vi "integrate_data view.vi"(8 "Y-column names":string[](array[string])=["col0"], 10 "column extension":string[](array[string])=["SCM1_2020Aug_AC.008.txt"], 11 "Graph array":cluster{"output":dbl[], "output":dbl[]}[](array[cluster])=[{"output"=array[591 elements], "output"=array[591 elements]}]) -> ()   [LabVIEW 2024]
uses:
  <vilib>/Analysis/2dsp.llb/Integral Method.ctl
  <vilib>/Analysis/1siggen.llb/Ramp Pattern by Samples.vi
  <vilib>/Analysis/NI_AALBase.lvlib
  <vilib>/gmath/NI_Gmath.lvlib
  <vilib>/Analysis/NI_AALPro.lvlib
panel:
  out "error code":i32
  out "bkg and subtracted data":cluster{"xi used":dbl[], "Integral X":dbl[]}[](graph)
  in  "remove bkg":bool=TRUE
  in  "Bbkg final":dbl=5.0 format="%.2f"
  in  "Bbkg initial":dbl=4.0 format="%.2f"
  in  "poly. order":i32=2
  in  "bkg removal method":enum16{"polynomial", "Cheby poly"}(ring)
  in  "integration method":T1=1 items=["Trapezoidal Rule", "Simpson's Rule", "Simpson's 3/8 Rule", "Bode Rule"]
  in  "export":T2(ring)=enum."write to clipboard"
  out "raw data/bkg":T3(graph)
  in  "interpol. method":i32(ring)=2 items=["nearest", "linear", "spline", "cubic Hermite", "Lagrange"]
  in  "stop":bool
  in  "use variables":bool
  in  "Interpolation #":i32=5000
  in  "export data":bool
  in  "smoothing factor":i32=1
  in  "final":dbl=5.0 format="%.2f"
  in  "init":dbl format="%.2f"
  out "integrated":cluster{"xi used":dbl[], "Integral X":dbl[]}[](graph)
  in  "variable":string="4.2\n3.5\n3"
  # "(0) Data are clipped defined by the 'init' and 'final'.\n(1) Boxcar averaging (use 'smoothing factor' for adjustment)\n(3) Background removal if necessary. Background removal is done by polynomial (normal or Chebychev).\n            i) fitting is done for the range given by 'Bbkg init' and 'Bbkg final'.\n            ii) the background curve is extended to the whole data range."
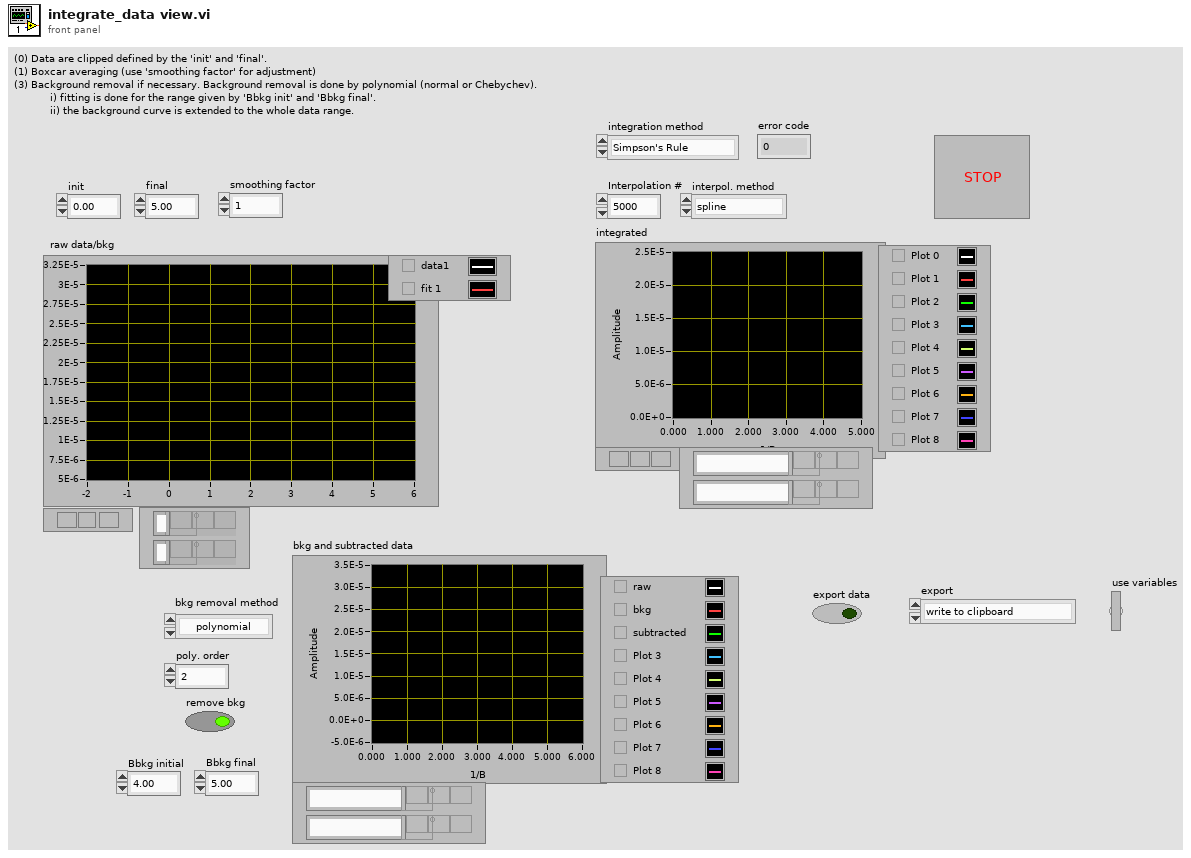
[diagram p1: front panel]
types:
  T1 = typedef "NI_AALPro.lvlib/Integral Method.ctl" = i32
  T2 = enum16{"Save as Ascill file", "write to clipboard", "write to Igor ITX file"}
  T3 = cluster{"Ramp Pattern":dbl[], "Power Spectrum":dbl[]}[]
  T4 = enum16{"Save as Ascill file", "write to clipboard", "do not export"}
  T5 = cluster{"all rows":dbl[], "extended data":dbl[]}[]
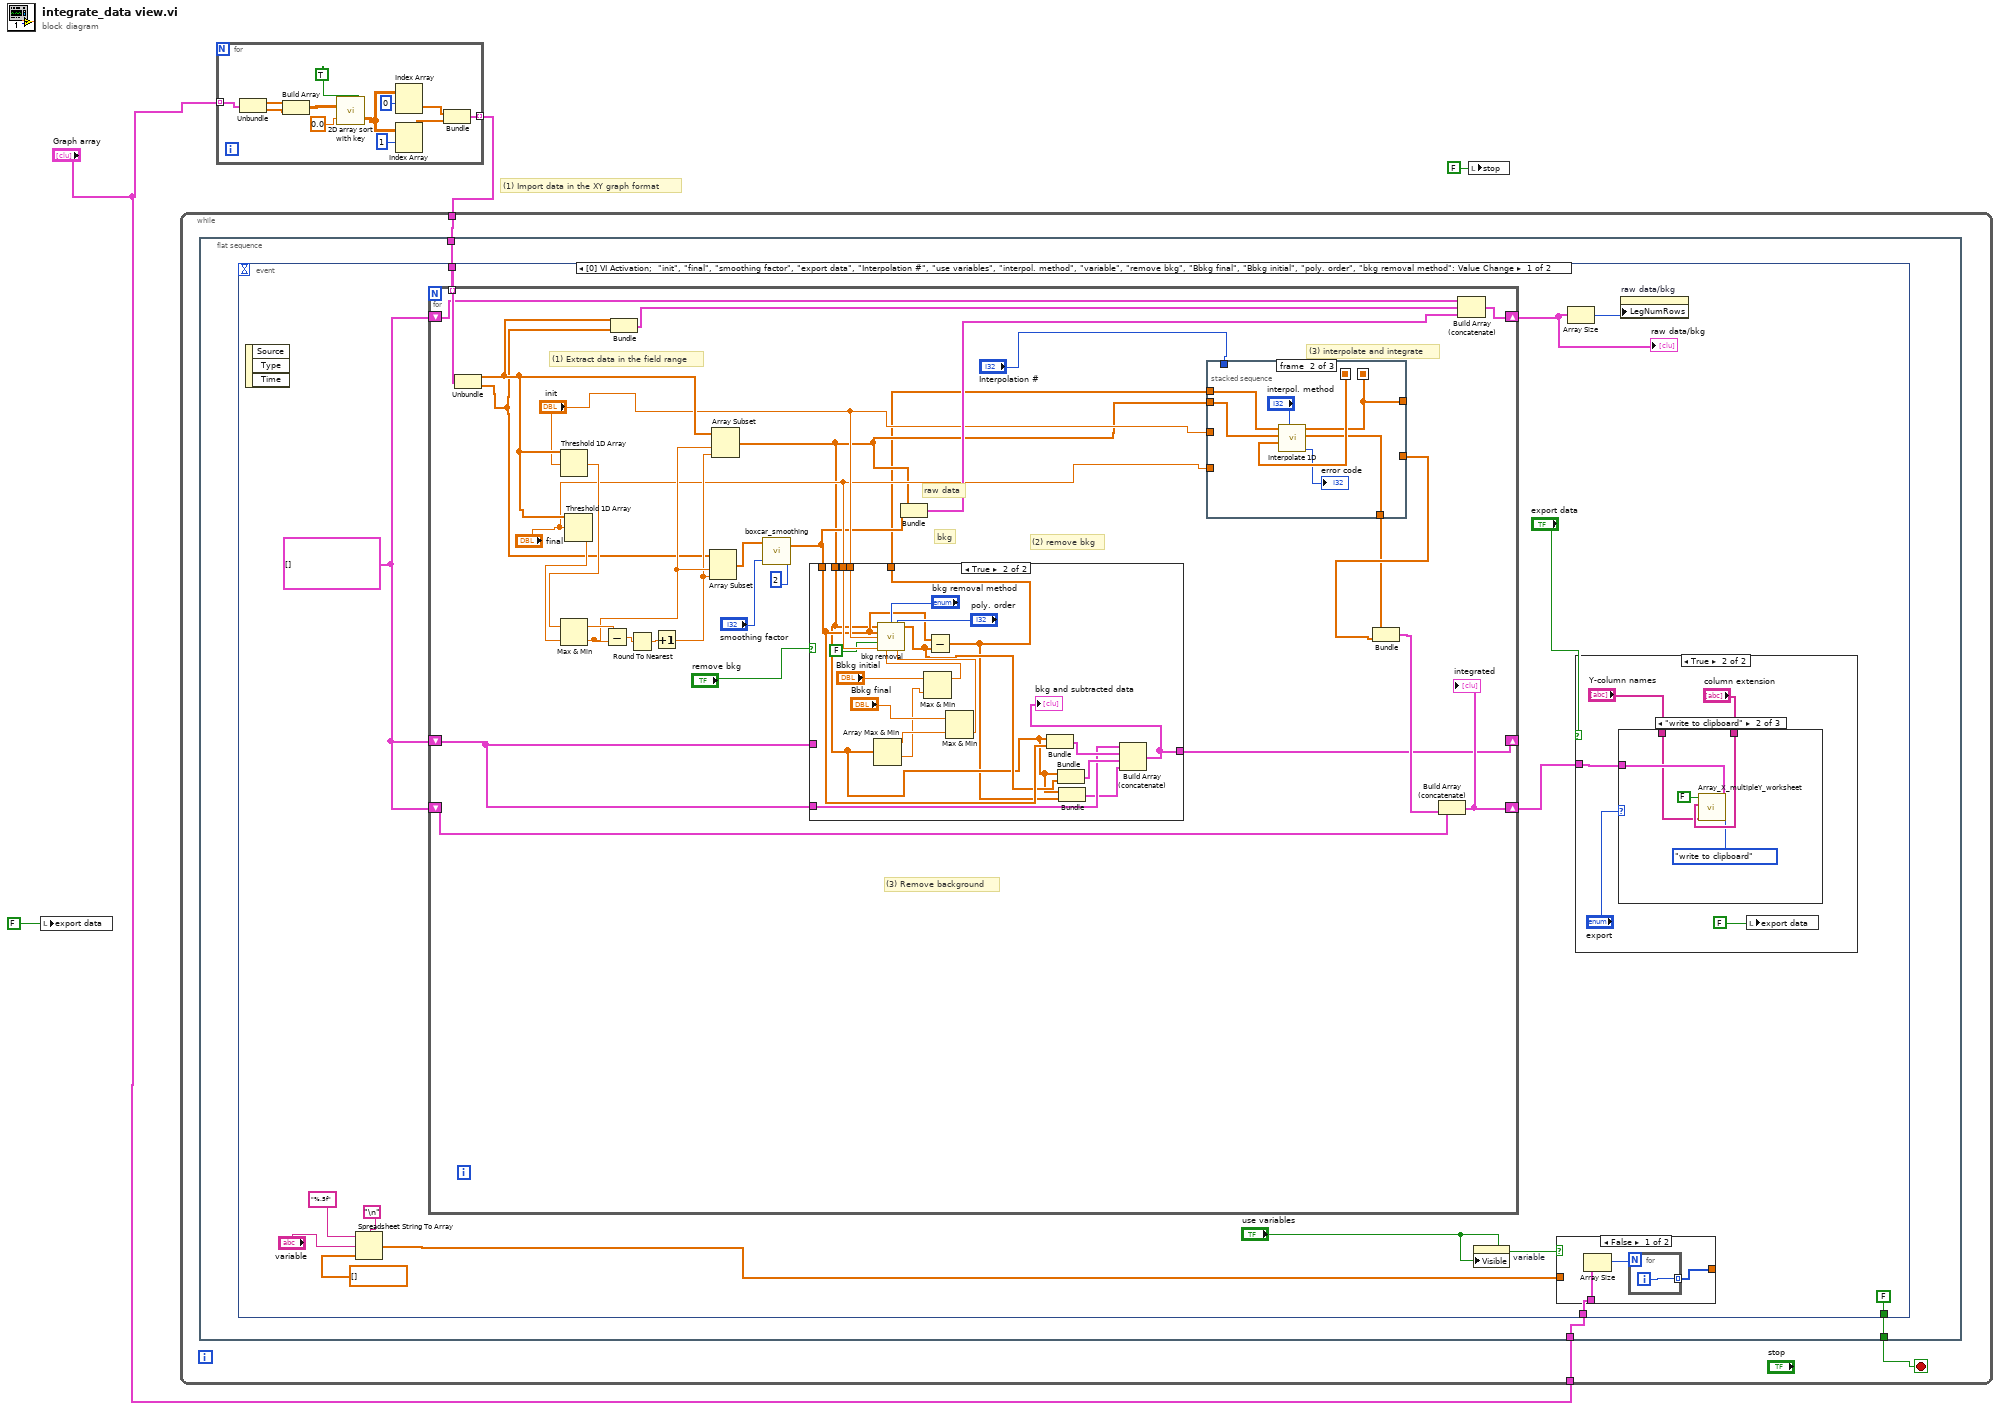
[diagram p0: block diagram]
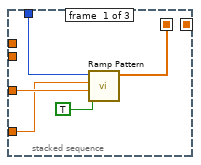
[diagram p4: hidden frame]
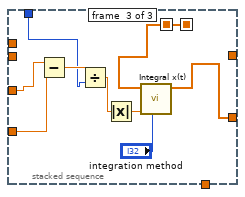
[diagram p5: hidden frame]
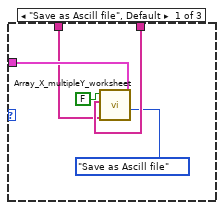
[diagram p7: hidden frame]
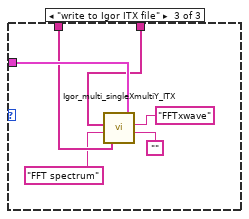
[diagram p8: hidden frame]
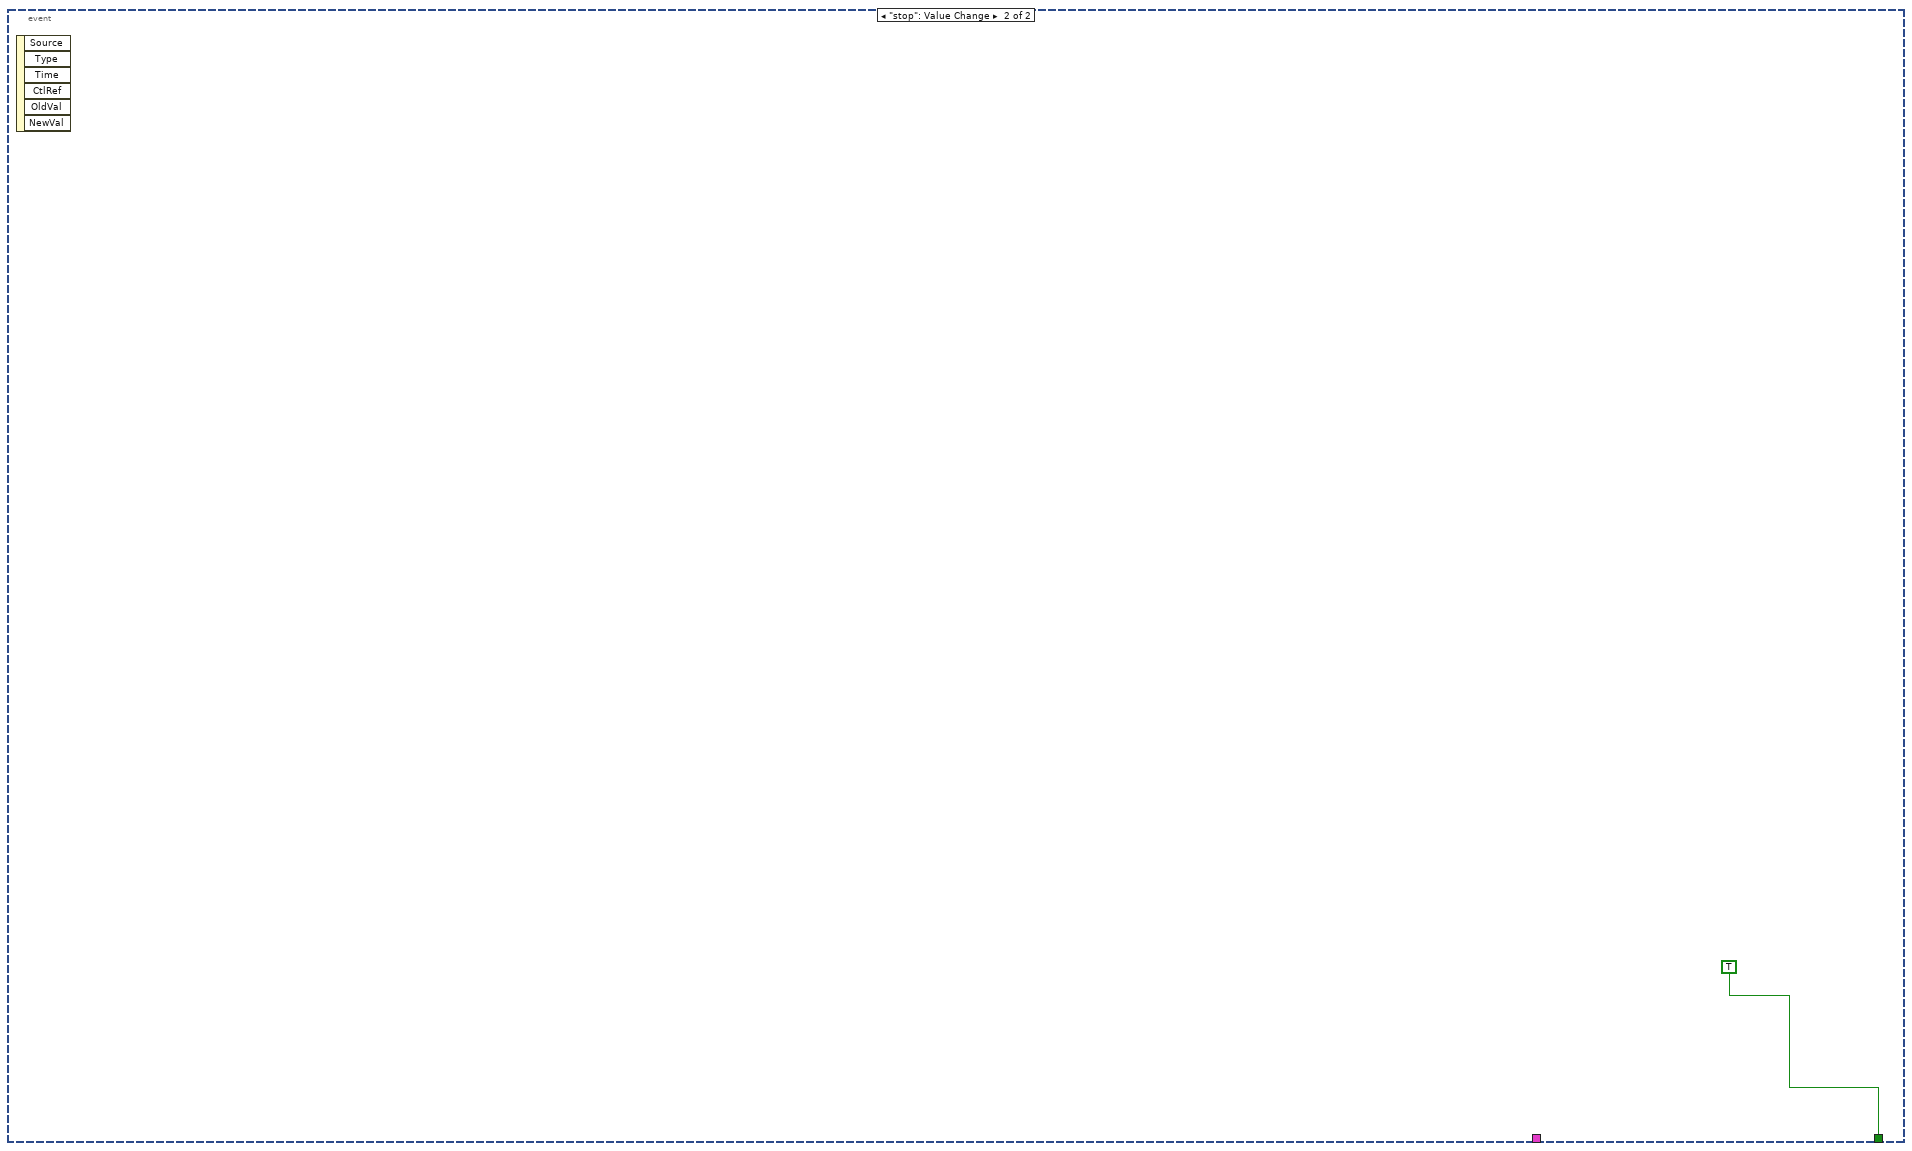
[diagram p9: hidden frame]
diagram:
  # "(1) Import data in the XY graph format"
  n1 = local write "export data"(FALSE ("export spectrum")) -> ()
  n2 = for {
    tunnel: "Graph array" -> [w16] mode=indexing
    tunnel: [w5] -> w3 mode=indexing
    n3 = Unbundle(w16) -> ("output"=w14:dbl[], "output"=w13:dbl[])
    n4 = Build Array(w14, w13) -> (w12:dbl[][])
    n5 = call "2D array sort with key.vi"("ascending"=TRUE, "key row"=0.0, "input"=w12) -> ("output"=w10:dbl[][])
    n6 = Index Array(array=w10, index (row)=0) -> (element=w7:dbl[])  [unwired: 1 in]
    n7 = Index Array(array=w10, index (row)=1) -> (element=w6:dbl[])  [unwired: 1 in]
    n8 = Bundle("output"=w7, "output"=w6) -> (w5:cluster{"output":dbl[], "output":dbl[]})  [unwired: 1 in]
  }
  n9 = while {
    tunnel: w3 -> [w19]
    tunnel: "Graph array" -> [w18]
    stop <- w17 stop-if-true
    n10 = flat-sequence {
      tunnel: w19 -> [w22]
      tunnel: w18 -> [w21]
      tunnel: [w20] -> w17
      frame #0 {
        n11 = event shown="[0] VI Activation;  \"init\", \"final\", \"smoothing factor\", \"export data\", \"Interpolation #\", \"use variables\", \"interpol. method\", \"variable\", \"remove bkg\", \"Bbkg final\", \"Bbkg initial\", \"poly. order\", \"bkg removal method\": Value Change" {
          selector: _ -> [_ _]
          dyn-events: _ -> [_ _]
          timeout: _ -> [_ _]
          tunnel: w22 -> [w31 _]
          tunnel: w21 -> [w29 _]
          tunnel: [FALSE ("stop (press twice)") TRUE ("stop (press twice)")] -> w20
          event VI Activation; "init", "final", "smoothing factor", "export data", "Interpolation #", "use variables", "interpol. method", "variable", "remove bkg", "Bbkg final", "Bbkg initial", "poly. order", "bkg removal method": Value Change {
            w23 = cluster{"all rows":sgl[], "all rows":sgl[]}[] []
            n12 = event-data() -> ()  [unwired: 1 in, 3 out]
            n13 = Spreadsheet String To Array(delimiter (Tab)="\n", format string="%.5f", spreadsheet string="variable", array type (2D Dbl)=dbl[] []) -> (array=w30:dbl[])
            n14 = for {
              shift-right: [w64] -> w24
              shift-left: w23 -> [w71]
              tunnel: w31 -> [w63] mode=indexing
              shift-right: [w61] -> w28
              shift-left: w23 -> [w60]
              shift-right: [w45] -> _
              shift-left: w23 -> [w44]
              # "(2) remove bkg"
              # "(3) interpolate and integrate"
              # "(3) Remove background"
              # "(1) Extract data in the field range"
              # "bkg"
              # "raw data"
              n15 = Unbundle(w63) -> ("output"=w59:dbl[], "output"=w56:dbl[])
              n16 = Threshold 1D Array(2:"init", 3:w59) -> (0:w70:dbl)  [unwired: 1 in]
              n17 = Threshold 1D Array(2:"final", 3:w59) -> (0:w69:dbl)  [unwired: 1 in]
              n18 = Max & Min(x=w70, y=w69) -> (max(x,y)=w68:dbl, min(x,y)=w66:dbl)
              n19 = Subtract(x=w68, y=w66) -> (x-y=w67:dbl)
              n20 = Bundle("output"=w59, "output"=w56) -> (w58:cluster{"output":dbl[], "output":dbl[]})  [unwired: 1 in]
              n21 = Round To Nearest(number=w67) -> (nearest integer value=w72:dbl)
              n22 = Increment(x=w72) -> (x+1=w65:dbl)
              n23 = Array Subset(array=w56, index=w66, length=w65) -> (w55:dbl[])
              n24 = Array Subset(array=w59, index=w66, length=w65) -> (w43:dbl[])
              n25 = call "boxcar_smoothing.vi"("iteration Number"=2, "smooth factor"="smoothing factor", "raw data"=w55) -> ("smoothed"=w46:dbl[])  [unwired: 1 in]
              n26 = case shown="True" "remove bkg" {
                tunnel: w43 -> [_ w77]
                tunnel: w46 -> [w74 w83]
                tunnel: "init" -> [_ w94]
                tunnel: "final" -> [_ w93]
                tunnel: [w74 w76] -> w42
                tunnel: [w73 w78] -> w45
                tunnel: w44 -> [_ w79]
                tunnel: w44 -> [w73 _]
                frame False {
                }
                frame True {
                  n27 = Array Max & Min(array=w77) -> (max value=w88:dbl, min value=w87:dbl)  [unwired: 2 out]
                  n28 = Max & Min(x="Bbkg initial", y=w87) -> (max(x,y)=w84:dbl)  [unwired: 1 out]
                  n29 = Max & Min(x="Bbkg final", y=w88) -> (min(x,y)=w85:dbl)  [unwired: 1 out]
                  n30 = call "bkg removal.vi"("Bfield"=w77, "bkg removal method"="bkg removal method", "poly. order"="poly. order", "Data"=w83, "B initial"=w94, "inverse"=FALSE, "B final"=w93, "Bbkg initial"=w84, "Bbkg final"=w85) -> ("extended data"=w82:dbl[])  [unwired: 4 in, 2 out]
                  n31 = Subtract(x=w83, y=w82) -> (x-y=w76:dbl[])
                  n32 = Bundle(w77, "smoothed"=w83) -> (w81:cluster{dbl[], "smoothed":dbl[]})  [unwired: 1 in]
                  n33 = Bundle(w77, "extended data"=w82) -> (w80:cluster{dbl[], "extended data":dbl[]})  [unwired: 1 in]
                  n34 = Bundle(w77, w76) -> (w75:cluster{dbl[], dbl[]})  [unwired: 1 in]
                  n35 = Build Array (concatenate)(w79, w81, w80, w75) -> (w78:T5)
                  "bkg and subtracted data" <- w78
                }
              }
              n36 = Bundle(w43, "smoothed"=w46) -> (w57:cluster{dbl[], "smoothed":dbl[]})  [unwired: 1 in]
              n37 = stacked-sequence {
                seq-local: [w95 _ _] -> [_ w104 _]
                seq-local: [_ w101 _] -> [_ _ w110]
                tunnel: w42 -> [_ w106 _]
                tunnel: w43 -> [_ w103 _]
                tunnel: "Interpolation #" -> [w99 _ w111]
                tunnel: "init" -> [w98 _ w114]
                tunnel: "final" -> [w97 _ w113]
                tunnel: [_ _ w108] -> w54
                tunnel: [_ w102 _] -> w51
                tunnel: [_ w101 _] -> _
                frame #0 {
                  n38 = call-poly <vilib>:"Ramp Pattern.vi"("exclude end?"=TRUE, "start"=w98, "end"=w97, "samples"=w99) -> ("Ramp Pattern"=w95:dbl[])  [unwired: 6 in, 1 out]
                }
                frame #1 {
                  n39 = call <vilib>:"Interpolate 1D.vi"("method"="interpol. method", "xi"=w104, "X"=w103, "Y"=w106) -> ("error"=→"error code":i32, "xi used"=w102:dbl[], "yi"=w101:dbl[])  [unwired: 5 in]
                }
                frame #2 {
                  n40 = Subtract(x=w114, y=w113) -> (x-y=w112:dbl)
                  n41 = Divide(x=w112, y=w111) -> (x/y=w109:dbl)
                  n42 = Absolute Value(x=w109) -> (abs(x)=w107:dbl)
                  n43 = call <vilib>:"Integral x(t).vi"("integration method"="integration method", "dt"=w107, "X"=w110) -> ("Integral X"=w108:dbl[])  [unwired: 7 in, 1 out]
                }
              }
              n44 = Bundle("xi used"=w51, "Integral X"=w54) -> (w50:cluster{"xi used":dbl[], "Integral X":dbl[]})  [unwired: 1 in]
              n45 = Build Array (concatenate)(w71, w50) -> (w64:cluster{"xi used":dbl[], "Integral X":dbl[]}[])
              "integrated" <- w64
              n46 = Build Array (concatenate)(w60, w58, w57) -> (w61:cluster{"output":dbl[], "smoothed":dbl[]}[])
            }
            "raw data/bkg" <- w28
            n47 = property on="variable" class="Str"("Visible"="use variables") -> ()  [unwired: 2 in, 2 out]
            n48 = case shown="False" "use variables" {
              tunnel: w30 -> [_ w41]
              tunnel: [w38 w41] -> _
              tunnel: w29 -> [w37 _]
              frame False {
                n49 = Array Size(array=w37) -> (size(s)=w39:i32)
                n50 = for {
                  N: w39 -> [_]
                  tunnel: [w40] -> w38 mode=indexing
                  i -> [w40]
                }
              }
              frame True {
              }
            }
            n51 = Array Size(array=w28) -> (size(s)=w27:i32)
            n52 = case shown="True" "export data" {
              tunnel: w24 -> [_ w119]
              frame False {
              }
              frame True {
                n53 = case shown="\"write to clipboard\"" "export" {
                  tunnel: w119 -> [w125 w130 w136]
                  tunnel: "column extension" -> [w123 w128 w135]
                  tunnel: "Y-column names" -> [w122 w127 w134]
                  frame "Save as Ascill file", Default {
                    n54 = call "Array_X_multipleY_worksheet.vi"("export"=T4."Save as Ascill file", "graph file"=w125, "Y-column names"=w122, "column extension"=w123, "Sort?"=FALSE) -> ()  [unwired: 3 in, 2 out]
                  }
                  frame "write to clipboard" {
                    n55 = call "Array_X_multipleY_worksheet.vi"("export"=T4."write to clipboard", "graph file"=w130, "Y-column names"=w127, "column extension"=w128, "Sort?"=FALSE) -> ()  [unwired: 3 in, 2 out]
                  }
                  frame "write to Igor ITX file" {
                    n56 = call "Igor_multi_singleXmultiY_ITX.vi"("message"="", "x-column name"="FFTxwave", "graph file"=w136, "Y-column names"=w134, "window name"="FFT spectrum", "column extension"=w135) -> ()  [unwired: 1 in, 1 out]
                  }
                }
                n57 = local write "export data"(FALSE ("export spectrum")) -> ()
              }
            }
            n58 = property on="raw data/bkg" class="XYGraph (strict)"("LegNumRows"=w27) -> ()  [unwired: 2 in, 2 out]
          }
          event "stop": Value Change {
            n59 = event-data() -> ()  [unwired: 1 in, 6 out]
          }
        }
      }
    }
  }
  n60 = local write "stop"(FALSE ("stop")) -> ()
